vi "GA Get Ext Di Bit.vi"(8 "error in (no error)":errorcluster caption="错误输入（无错误）", 9 "pValue":u16, 10 "nBitIndex":i16, 11 "nCardIndex":i16) -> (0 "error out":errorcluster caption="错误输出", 1 "pValue out":u16, 3 "function return":i32)   [LabVIEW 2015, in "GAS.lvlib"]
doc: "extern \"C\" __declspec(dllimport) int GA_GetExtDiBit(short nCardIndex,short nBitIndex,unsigned short *pValue);"
uses:
  <userlib>/BP_GAS/GAS.lvlib
  <userlib>/BP_GAS/GAS.dll
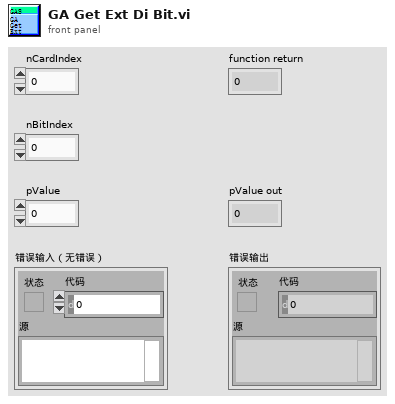
[diagram p1: front panel]
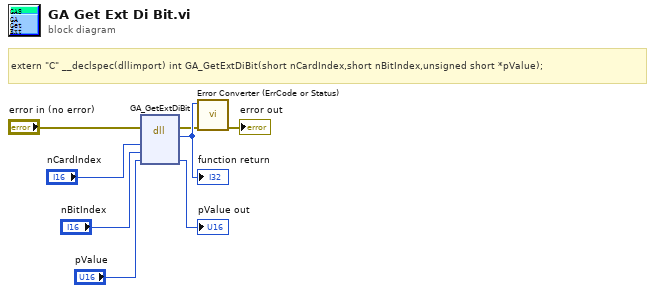
[diagram p0: block diagram]
diagram:
  # "extern \"C\" __declspec(dllimport) int GA_GetExtDiBit(short nCardIndex,short nBitIndex,unsigned short *pValue);"
  n1 = dll-call lib="E:/Program Files (x86)/National Instruments/LabVIEW 2015/user.lib/BP_GAS/GAS.*" fn="GA_GetExtDiBit"(error in="error in (no error)", "nCardIndex"="nCardIndex", "nBitIndex"="nBitIndex", "pValue"="pValue") -> (error out=w2:errorcluster, w8:i32, "pValue"=→"pValue out":u16)  [unwired: 4 in, 1 out]
  "function return" <- w8
  n2 = call "Error Converter (ErrCode or Status).vi"("error in (no error)"=w2, "error code"=w8) -> ("error out"=→"error out":errorcluster)  [unwired: 9 in]
